vi "String Search Speed.vi"() -> ()   [LabVIEW 2016]
panel:
  out "Array":string[](array[string])
  out "Attribute Search":u32
  out "Array Serach":u32
  out "found":bool
  out "index of element":i32
  in  "Numeric":i32=10000
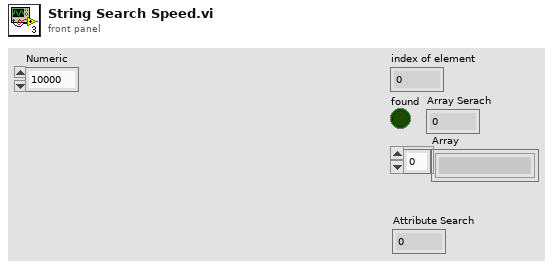
[diagram p1: front panel]
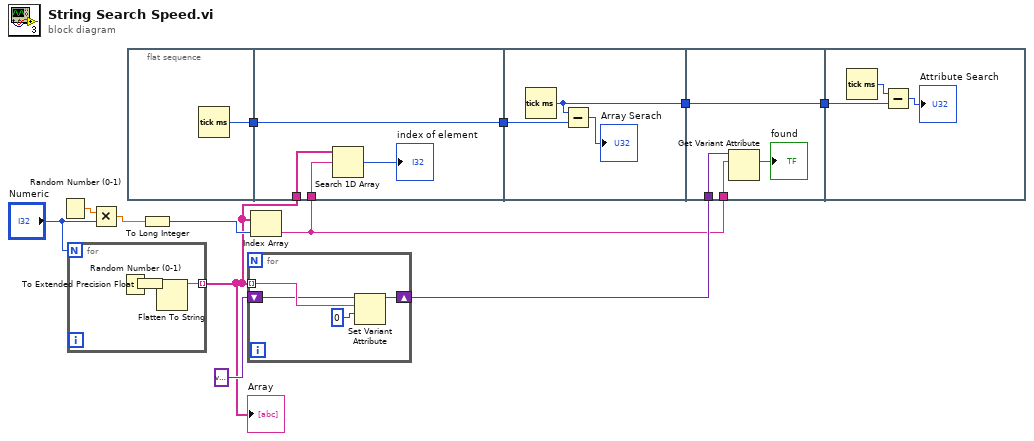
[diagram p0: block diagram]
diagram:
  n1 = Random Number (0-1)() -> (number: 0 to 1=w11:dbl)
  n2 = for {
    N: "Numeric" -> [_]
    tunnel: [w14] -> w7 mode=indexing
    n3 = Random Number (0-1)() -> (number: 0 to 1=w15:dbl)
    n4 = To Extended Precision Float(1:w15) -> (0:w13:ext)
    n5 = Flatten To String(anything=w13) -> (data string=w14:string)  [unwired: 3 in, 2 out]
  }
  "Array" <- w7
  n6 = Multiply(x=w11, y="Numeric") -> (x*y=w9:dbl)
  n7 = flat-sequence {
    tunnel: [w16] -> w4
    tunnel: w7 -> [w20]
    tunnel: w5 -> [w19]
    tunnel: w4 -> [w17]
    tunnel: [w17] -> w3
    tunnel: w3 -> [w23]
    tunnel: [w22] -> w2
    tunnel: w6 -> [w27]
    tunnel: w5 -> [w26]
    tunnel: w2 -> [w24]
    tunnel: [w24] -> w1
    tunnel: w1 -> [w29]
    frame #0 {
      n8 = Tick Count (ms)() -> (millisecond timer value=w16:u32)
    }
    frame #1 {
      n9 = Search 1D Array(1D array=w20, element=w19) -> (index of element=→"index of element":i32)  [unwired: 1 in]
    }
    frame #2 {
      n10 = Tick Count (ms)() -> (millisecond timer value=w22:u32)
      n11 = Subtract(x=w22, y=w23) -> (x-y=→"Array Serach":u32)
    }
    frame #3 {
      n12 = Get Variant Attribute(Variant=w27, name=w26) -> (found=→"found":bool)  [unwired: 2 in, 3 out]
    }
    frame #4 {
      n13 = Tick Count (ms)() -> (millisecond timer value=w30:u32)
      n14 = Subtract(x=w30, y=w29) -> (x-y=→"Attribute Search":u32)
    }
  }
  n15 = To Long Integer(number=w9) -> (32bit integer=w8:i32)
  n16 = for {
    tunnel: w7 -> [w34] mode=indexing
    shift-right: [w33] -> w6
    shift-left: variant -> [w32]
    n17 = Set Variant Attribute(Variant=w32, name=w34, value=0) -> (Variant out=w33:variant)  [unwired: 1 in, 2 out]
  }
  n18 = Index Array(array=w7, index=w8) -> (element=w5:string)
